vi "53_RC Servo Motor_speed.vi"() -> ()   [LabVIEW 2018]
uses:
  <userlib>/KNR OS 4.0 LabVIEW Toolkit/Type Definition/Resource.ctl
  <userlib>/KNR OS 4.0 LabVIEW Toolkit/Type Definition/RC Servo Port.ctl
panel:
  in  "millisecond multiple":u32(slide)=50 scale=10.0..100.0
  in  "stop":bool
  # "700~2300"
  # "295~2652"
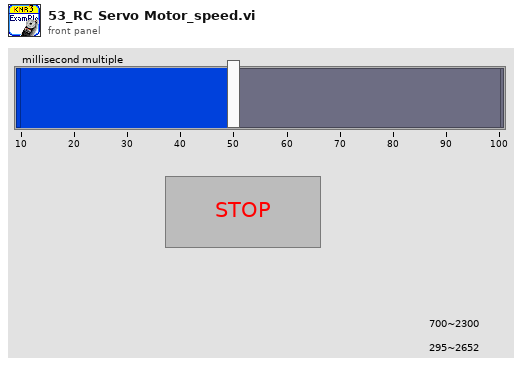
[diagram p1: front panel]
types:
  T1 = typedef "Resource.ctl" = enum16{"KNRm_DDRC", "KNRm_DDDD", "KNRm_DDDR", "KNRm_DDDC", "KNR", "KNRm_neww"}
  T2 = typedef "KNR3 Reference.ctl" = cluster{"FPGA Session":refnum<class "FPGA Interface Base.lvclass">, "Resource":T1}
  T3 = typedef "RC Servo Port.ctl" = u16
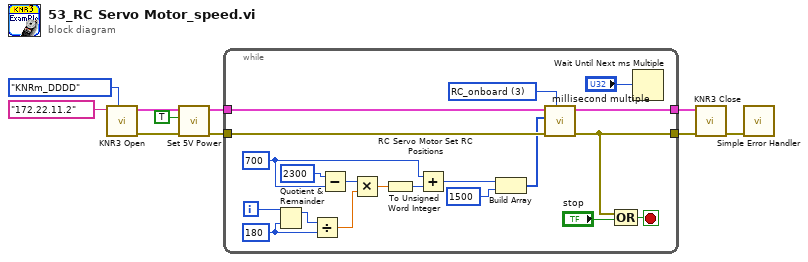
[diagram p0: block diagram]
diagram:
  n1 = call <userlib>:"KNR3 Open.vi"("Resource"=Resource."KNRm_DDDD", "IP"="172.22.11.2") -> ("error out"=w8:errorcluster, "KNR out"=w10:T2)  [unwired: 8 in]
  n2 = call <userlib>:"Set 5V Power.vi"("error in (no error)"=w8, "5V Power(T)"=TRUE ("5V Power"), "KNR in"=w10) -> ("error out"=w7:errorcluster, "KNR out"=w9:T2)  [unwired: 7 in]
  n3 = while {
    tunnel: w9 -> [w30]
    tunnel: [w29] -> w2
    tunnel: w7 -> [w28]
    tunnel: [w25] -> w1
    i -> [w15]
    stop <- w27 stop-if-true
    w22 = u16 700
    w20 = u16 180 ("y")
    w24 = T3 3 items=["RC_onboard"=3, "RC_box"=9] ("RC Motor")
    n4 = Quotient & Remainder(x=w15, y=w20) -> (x-y*floor(x/y)=w21:i32)  [unwired: 1 out]
    n5 = Divide(x=w21, y=w20) -> (x/y=w18:dbl)
    n6 = Subtract(x=u16 2300, y=w22) -> (x-y=w19:u16)
    n7 = Multiply(x=w19, y=w18) -> (x*y=w17:dbl)
    n8 = To Unsigned Word Integer(number=w17) -> (unsigned 16bit integer=w16:u16)
    n9 = Add(x=w22, y=w16) -> (x+y=w12:u16)
    n10 = Build Array(w12, u16 1500) -> (w14:u16[])
    n11 = call <userlib>:"RC Servo Motor Set RC Positions.vi"("Port (RC_onboard)"=w24, "error in (no error)"=w28, "RC Pulse Width (1500 uS)"=w14, "KNR in"=w30) -> ("error out"=w25:errorcluster, "KNR out"=w29:T2)  [unwired: 6 in]
    n12 = Compound Arithmetic op=OR(w25, "stop") -> (w27:bool)
    n13 = Wait Until Next ms Multiple(millisecond multiple="millisecond multiple") -> ()  [unwired: 1 out]
  }
  n14 = call <userlib>:"KNR3 Close.vi"("error in (no error)"=w1, "KNR in"=w2) -> ("error out"=w6:errorcluster)  [unwired: 9 in]
  n15 = call <vilib>:"Simple Error Handler.vi"("error in (no error)"=w6) -> ()  [unwired: 4 in, 5 out]
